vi "SaveRefs.vi"(7 "error in":errorcluster, 9 "Références à charger":dbl[][](array[numeric]), 10 "file path (use dialog)":path) -> (0 "error out":errorcluster)   [LabVIEW 2013]
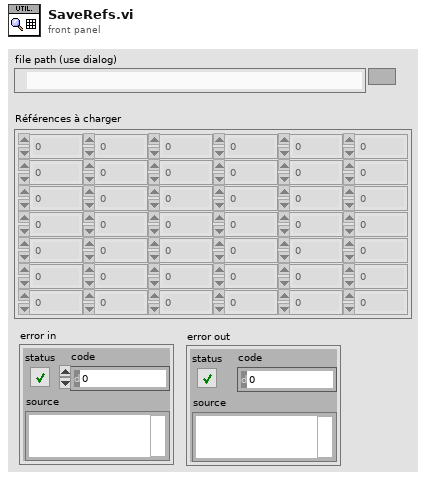
[diagram p1: front panel]
types:
  T1 = enum16{"open", "replace", "create", "open or create", "replace or create", "replace or create with confirmation"}
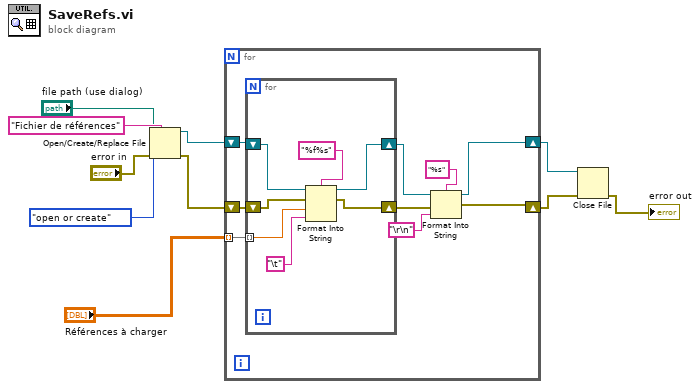
[diagram p0: block diagram]
diagram:
  n1 = Open/Create/Replace File(file path (use dialog)="file path (use dialog)", error in="error in", prompt="Fichier de références", operation (0:open)=T1."open or create") -> (refnum out=w6:refnum<file>, error out=w7:errorcluster)  [unwired: 2 in, 1 out]
  n2 = for {
    tunnel: "Références à charger" -> [w19] mode=indexing
    shift-right: [w12] -> w4
    shift-left: w7 -> [w18]
    shift-right: [w13] -> w5
    shift-left: w6 -> [w16]
    n3 = for {
      tunnel: w19 -> [w25] mode=indexing
      shift-right: [w22] -> w17
      shift-left: w18 -> [w23]
      shift-right: [w20] -> w15
      shift-left: w16 -> [w21]
      n4 = Format Into String(format string="%f%s", initial string=w21, error in=w23, w25, "\t") -> (resulting string=w20:refnum<file>, error out=w22:errorcluster)
    }
    n5 = Format Into String(format string="%s", initial string=w15, error in=w17, "\r\n") -> (resulting string=w13:refnum<file>, error out=w12:errorcluster)
  }
  n6 = Close File(refnum=w5, error in=w4) -> (error out=→"error out":errorcluster)  [unwired: 1 out]
